vi "lireresultat.vi"() -> (0 "etat de marquage":string)   [LabVIEW 2021]
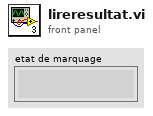
[diagram p1: front panel]
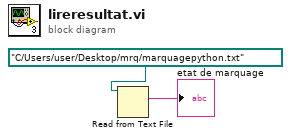
[diagram p0: block diagram]
diagram:
  n1 = Read from Text File(file (use dialog)=path "C:/Users/user/Desktop/mrq/marquagepython.txt" ("file path (dialog if empty)")) -> (text=→"etat de marquage":string)  [unwired: 3 in, 3 out]
